vi "Create Cluster.vi"(8 "error in (no error)":errorcluster, 10 "Cluster Name":string, 11 "System in":refnum<class "System.lvclass">) -> (0 "error out":errorcluster, 2 "Cluster":refnum<class "Cluster.lvclass">, 3 "System out":refnum<class "System.lvclass">)   [LabVIEW 2020, in "VolatusConfig.lvlib" / "System.lvclass"]
uses:
  System.lvclass
  System.lvclass/System.ctl
  VolatusConfigElement/VolatusConfigElement.lvclass
  Cluster/Cluster.lvclass
  lv-cdm/CDM-Config/Config Element/Config Element.lvclass
  C:/dev/lv20CE/relink/lv-volatus/VolatusConfig/VolatusConfigElement/VolatusConfigElement.lvclass
  C:/dev/lv20CE/relink/lv-volatus/VolatusConfig/System/System.lvclass
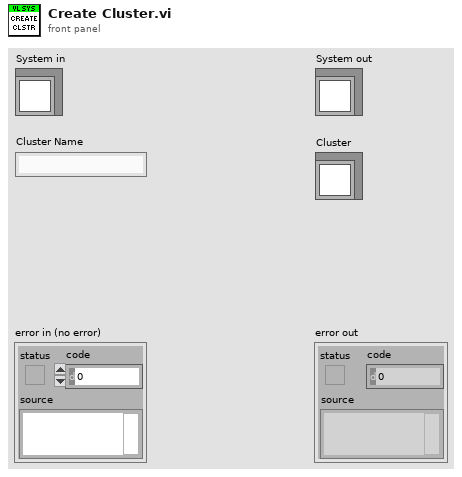
[diagram p1: front panel]
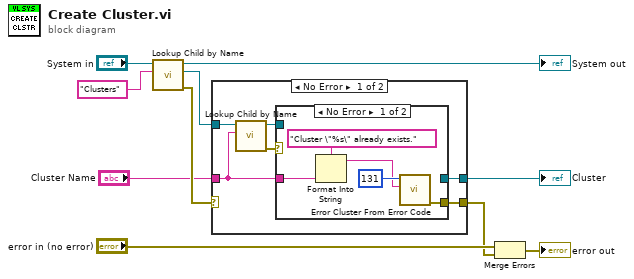
[diagram p0: block diagram]
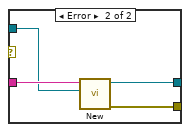
[diagram p2: hidden frame]
diagram:
  n1 = call "Lookup Child by Name.vi"("Child Name"="Clusters", "VolatusConfigElement in"="System in") -> ("error out"=w10:errorcluster, "Child"=w1:refnum<class "Config Element.lvclass">, "VolatusConfigElement out"=→"System out":refnum<class "System.lvclass">)  [unwired: 6 in, 1 out]
  n2 = case shown="No Error" w10 {
    selector: w10 -> [_ w26]
    tunnel: "Cluster Name" -> [w13 _]
    tunnel: [w16 w26] -> w3
    tunnel: [w15 _] -> w2
    tunnel: w1 -> [w14 _]
    frame No Error {
      n3 = call "Lookup Child by Name.vi"("Name"=w13, "Config Element in"=w14) -> ("error out"=w11:errorcluster, "Config Element out"=w12:refnum<class "Config Element.lvclass">)  [unwired: 6 in, 2 out]
      n4 = case shown="No Error" w11 {
        tunnel: [w21 w25] -> w16
        tunnel: [_ w24] -> w15
        tunnel: w13 -> [w18 w23]
        tunnel: w12 -> [_ w22]
        frame No Error {
          n5 = Format Into String(format string="Cluster \"%s\" already exists.", w18) -> (resulting string=w17:string)  [unwired: 2 in, 1 out]
          n6 = call <vilib>:"Error Cluster From Error Code.vi"("error message (\"\")"=w17, "error code (0)"=131) -> ("error out"=w21:errorcluster)  [unwired: 7 in]
        }
        frame Error {
          n7 = call "New.vi"("Parent"=w22, "Name"=w23) -> ("error out"=w25:errorcluster, "Cluster out"=w24:refnum<class "Cluster.lvclass">)  [unwired: 8 in]
        }
      }
    }
    frame Error {
    }
  }
  "Cluster" <- w2
  n8 = Merge Errors("error in (no error)", w3) -> (→"error out":errorcluster)
